vi "Async OIM Data.vi"(8 "error in (no error)":errorcluster, 10 "Address":u8=4, 11 "Modbus Master in":refnum<class "Modbus Master.lvclass">) -> (0 "error out":errorcluster, 2 "Resistance 2":dbl, 3 "Modbus Master out":refnum<class "Modbus Master.lvclass">, 5 "Insulation Fault_24V":bool)   [LabVIEW 2024]
uses:
  <vilib>/Modbus/master/Modbus Master.lvclass
  C:/Program Files (x86)/National Instruments/LabVIEW 2024/vi.lib/Modbus/subvis/Modbus API/Modbus API.lvclass
  <vilib>/Modbus/subvis/Modbus API/Modbus API.lvclass/Modbus API.ctl
  <vilib>/Modbus/subvis/Transmission Data Unit (ADU)/Transmission Data Unit/Transmission Data Unit.lvclass/Transmission Data Unit.ctl
  <vilib>/Modbus/master/Data Access/Unit ID/Set Unit ID Property.vi
  <vilib>/Modbus/subvis/Transmission Data Unit (ADU)/Transmission Data Unit/Data Access/Unit ID/Write Unit ID.vi
  <vilib>/Modbus/subvis/Modbus API/Read Transmission Data Unit.vi
  <vilib>/Modbus/subvis/Modbus API/Write Transmission Data Unit.vi
  <vilib>/Modbus/subvis/Transmission Data Unit (ADU)/Transmission Data Unit/Transmission Data Unit.lvclass
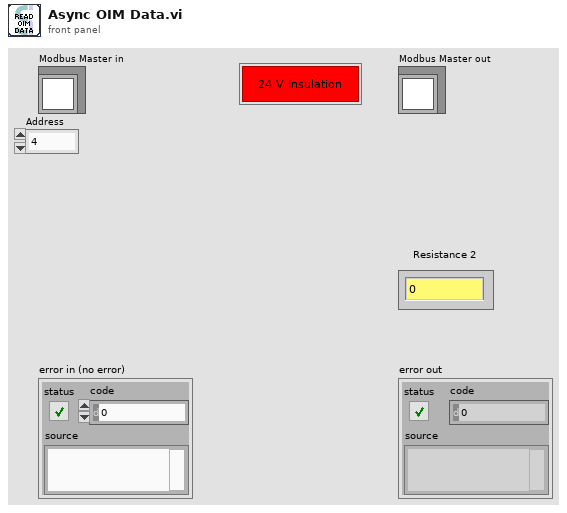
[diagram p1: front panel]
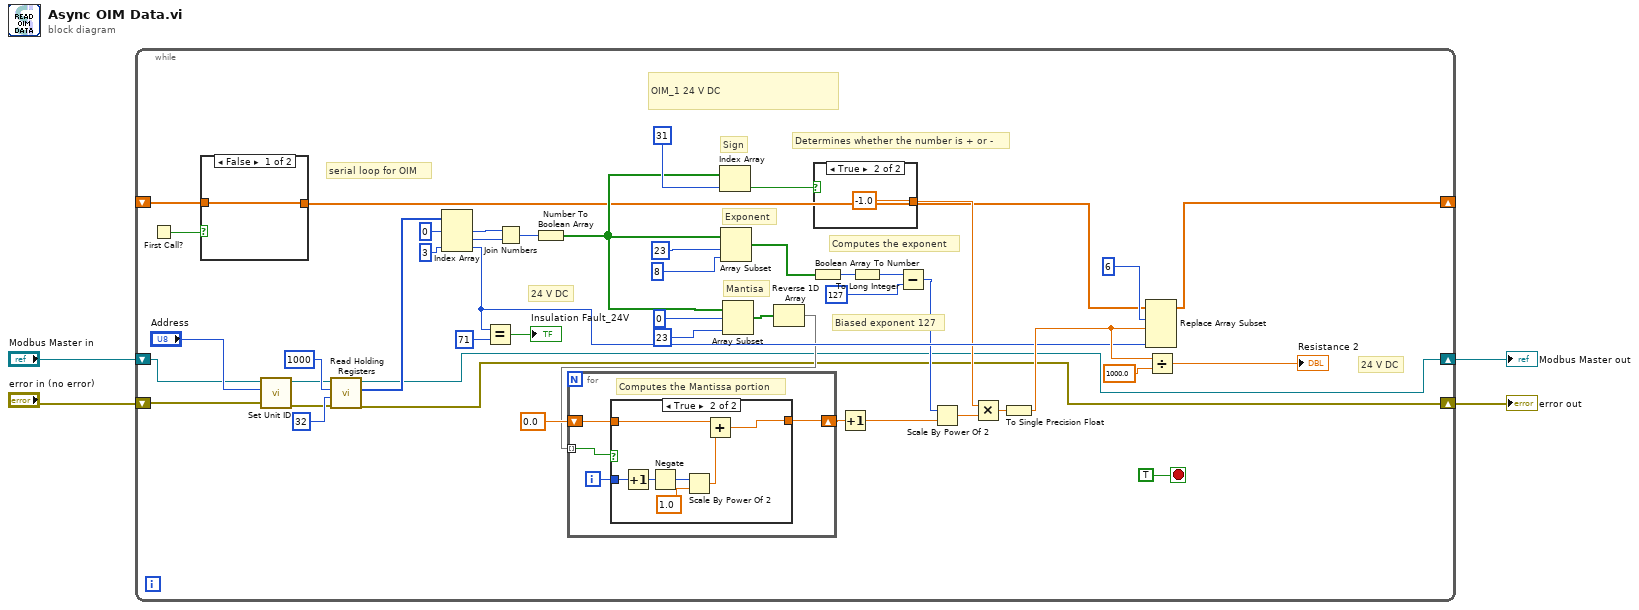
[diagram p0: block diagram]
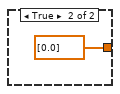
[diagram p2: hidden frame]
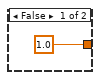
[diagram p3: hidden frame]
diagram:
  n1 = while {
    shift-right: [w11] -> _
    shift-left: _ -> [w6]
    shift-right: [w9] -> w3
    shift-left: "Modbus Master in" -> [w12]
    shift-right: [w10] -> w4
    shift-left: "error in (no error)" -> [w13]
    stop <- TRUE stop-if-true
    # "24 V DC"
    # "24 V DC"
    # "OIM_1 24 V DC"
    # "serial loop for OIM"
    # "Biased exponent 127"
    # "Mantisa"
    # "Exponent"
    # "Sign"
    # "Computes the exponent"
    # "Determines whether the number is + or -"
    n2 = First Call?() -> (First Call?: T/F=w5:bool)
    n3 = case shown="False" w5 {
      tunnel: [w52 sgl[] [0.0]] -> w7
      tunnel: w6 -> [w52 _]
      frame False {
      }
      frame True {
      }
    }
    n4 = call <vilib>:"Set Unit ID.vi"("error in (no error)"=w13, "unit ID"="Address", "Modbus master in"=w12) -> ("error out"=w47:errorcluster, "Modbus master out"=w48:refnum<class "Modbus Master.lvclass">)  [unwired: 7 in]
    n5 = call-dynamic "Read Holding Registers.vi"("error in (no error)"=w47, "number of holding registers"=u16 32, "starting address"=u16 1000, "Modbus master in"=w48) -> ("error out"=w10:errorcluster, "register values"=w45:u16[], "Modbus master out"=w9:refnum<class "Modbus Master.lvclass">)  [unwired: 5 in]
    n6 = Index Array(array=w45, index #1=0 ("index"), index #3=3 ("index")) -> (element #1=w16:u16, element #2=w17:u16, element #3=w41:u16)  [unwired: 1 in]
    n7 = Equal?(x=w41, y=u16 71) -> (x = y?=→"Insulation Fault_24V":bool)
    n8 = Join Numbers(hi=w16, lo=w17) -> ((hi.lo)=w15:u32)
    n9 = Number To Boolean Array(number=w15) -> (Boolean array=w14:bool[])
    n10 = Index Array(array=w14, index=31) -> (element=w25:bool)
    n11 = Array Subset(array=w14, index=23, length=8) -> (w24:bool[])
    n12 = Array Subset(array=w14, index=0, length=23) -> (w23:bool[])
    n13 = Reverse 1D Array(array=w23) -> (reversed array=w22:bool[])
    n14 = for {
      tunnel: w22 -> [w59] mode=indexing
      shift-right: [w56] -> w34
      shift-left: 0.0 -> [w57]
      i -> [w58]
      # "Computes the Mantissa portion"
      n15 = case shown="True" w59 {
        tunnel: w58 -> [_ w67]
        tunnel: w57 -> [w60 w63]
        tunnel: [w60 w61] -> w56
        frame False {
        }
        frame True {
          n16 = Increment(x=w67) -> (x+1=w66:i32)
          n17 = Negate(x=w66) -> (-x=w65:i32)
          n18 = Scale By Power Of 2(n=w65, x=1.0) -> (x*2^n=w62:dbl)
          n19 = Add(x=w63, y=w62) -> (x+y=w61:dbl)
        }
      }
    }
    n20 = Boolean Array To Number(Boolean array=w24) -> (number=w27:u32)
    n21 = case shown="True" w25 {
      tunnel: [1.0 -1.0] -> w29
      frame False {
      }
      frame True {
      }
    }
    n22 = Increment(x=w34) -> (x+1=w32:dbl)
    n23 = To Long Integer(number=w27) -> (32bit integer=w26:i32)
    n24 = Subtract(x=w26, y=127) -> (x-y=w28:i32)
    n25 = Scale By Power Of 2(n=w28, x=w32) -> (x*2^n=w31:dbl)
    n26 = Multiply(x=w29, y=w31) -> (x*y=w30:dbl)
    n27 = To Single Precision Float(number=w30) -> (single precision float=w43:sgl)
    n28 = Replace Array Subset(array=w7, new element #1=w43, index #1=6 ("index"), new element #2=w41) -> (w11:sgl[])  [unwired: 1 in]
    n29 = Divide(x=w43, y=sgl 1000.0) -> (x/y=→"Resistance 2":sgl)
  }
  "error out" <- w4
  "Modbus Master out" <- w3
